vi "Set Menu Items.vi"(8 "error in":errorcluster, 11 "History":refnum<class "History.lvclass">) -> (0 "error out":errorcluster)   [LabVIEW 2020, in "lv_icon.lvlib" / "History.lvlib" / "History.lvclass"]
doc: "Enables or disables the Redo and Undo menu items based on the Available Undo and Available Redo."
uses:
  History.lvclass
  History.lvclass/History.ctl
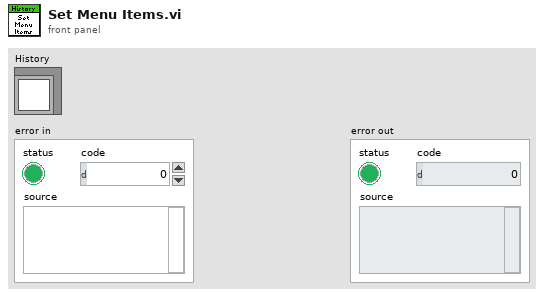
[diagram p1: front panel]
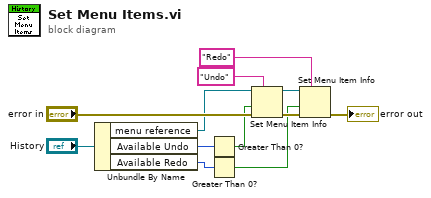
[diagram p0: block diagram]
diagram:
  n1 = Unbundle By Name("History") -> ("menu reference"=w3:refnum<k9>, "Available Undo"=w2:i32, "Available Redo"=w1:i32)
  n2 = Greater Than 0?(x=w2) -> (x > 0?=w9:bool)
  n3 = Greater Than 0?(x=w1) -> (x > 0?=w8:bool)
  n4 = Set Menu Item Info(7:"Undo" ("Redo Menu Item"), 8:"error in", 9:w9, 11:w3) -> (0:w12:errorcluster, 3:w7:refnum<k9>)  [unwired: 3 out]
  n5 = Set Menu Item Info(7:"Redo" ("Undo Menu Item"), 8:w12, 9:w8, 11:w7) -> (0:→"error out":errorcluster)  [unwired: 4 out]
